vi "main.vi"() -> ()   [LabVIEW 2023]
panel:
  out "Fall Time":dbl format="%#_6ps"
  in  "Stop":bool
  in  "Start":bool
  out "Error_Out":errorcluster
  in  "Amplitude(V)":dbl=5.0
  out "Digital Signal":i32[](graph)
  out "Rise time":dbl format="%#_6ps"
  out "min value":dbl format="%#_3g V"
  out "max value":dbl format="%#_3g V"
  in  "Error_In":errorcluster
  out "Square Wave":waveform(dbl)(graph)={"t0"=timestamp(0 s since 1904-01-01), "dt"=1e-06, "Y"=array[5000 elements]}
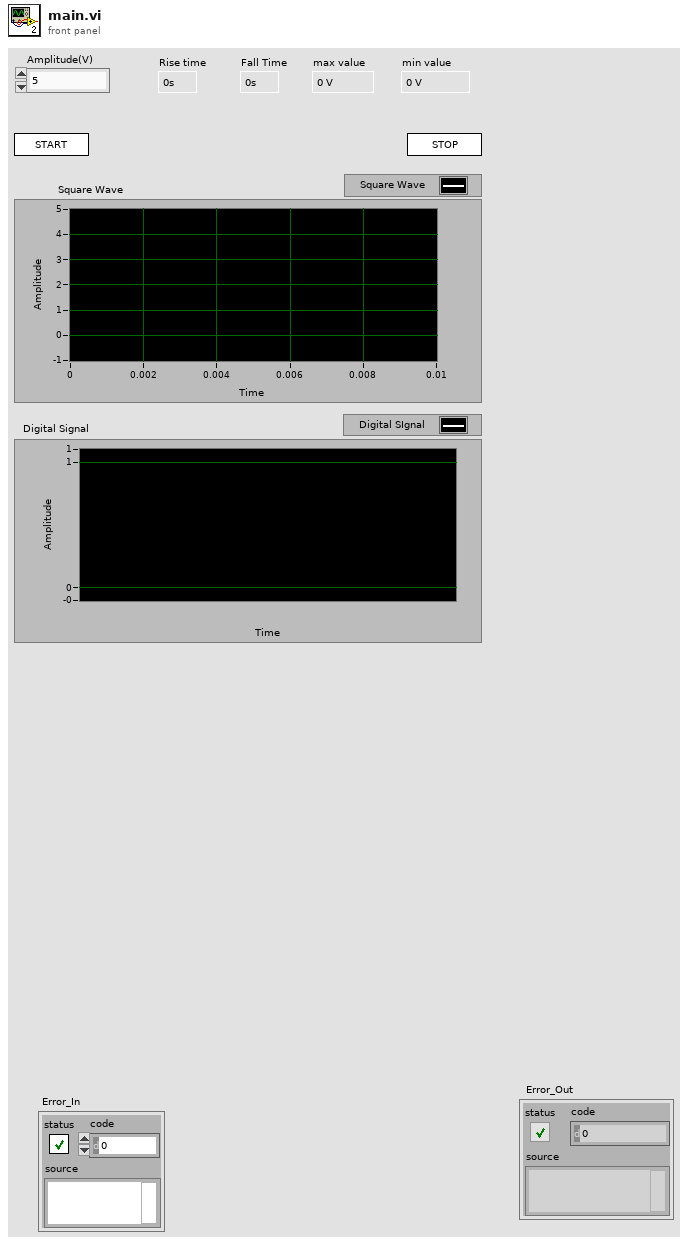
[diagram p1: front panel]
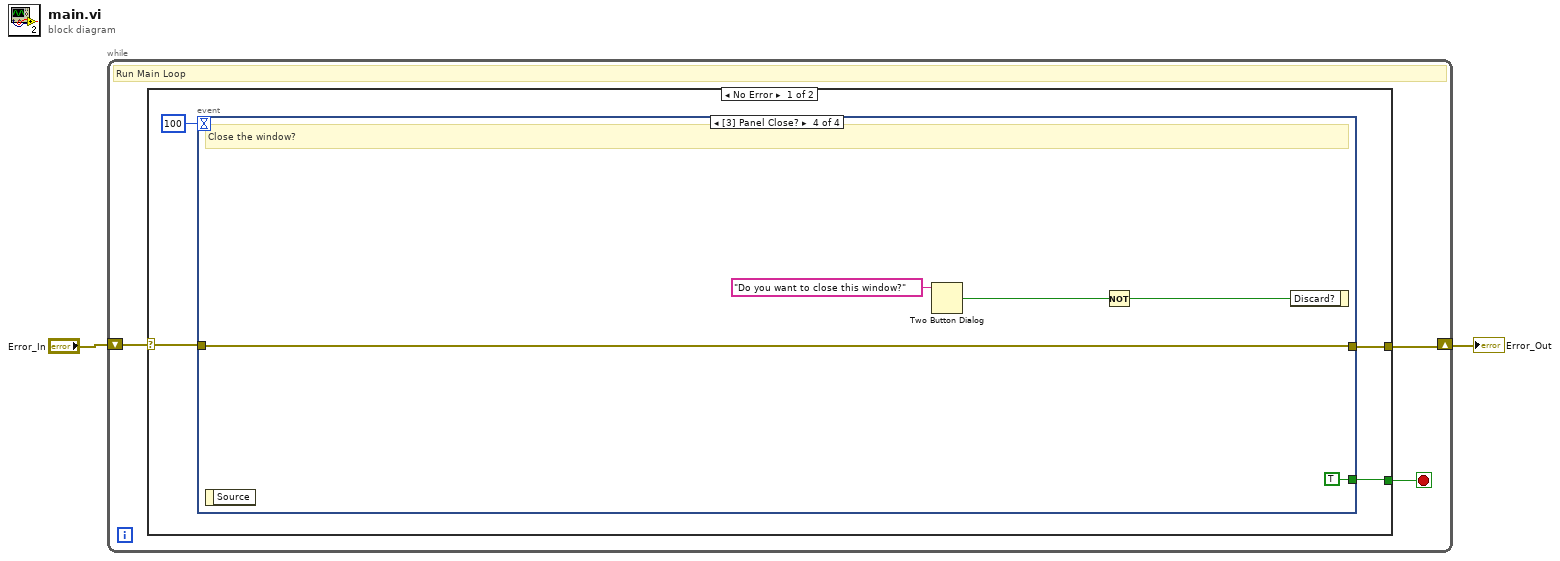
[diagram p0: block diagram]
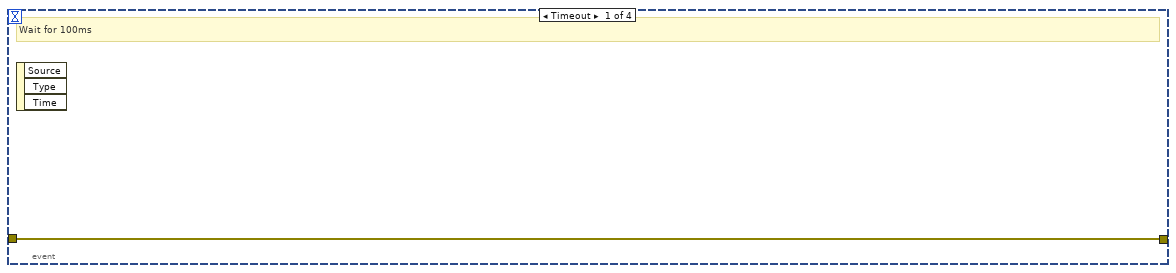
[diagram p2: hidden frame]
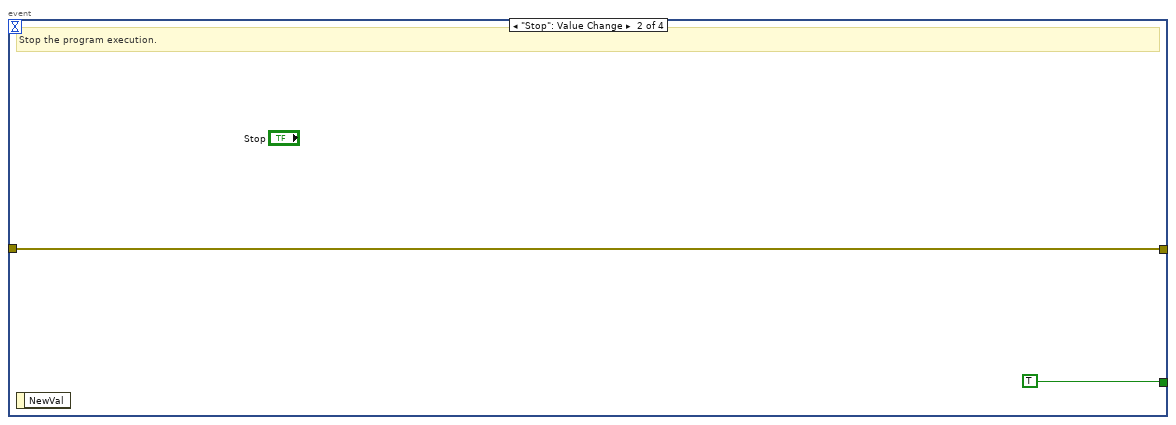
[diagram p3: hidden frame]
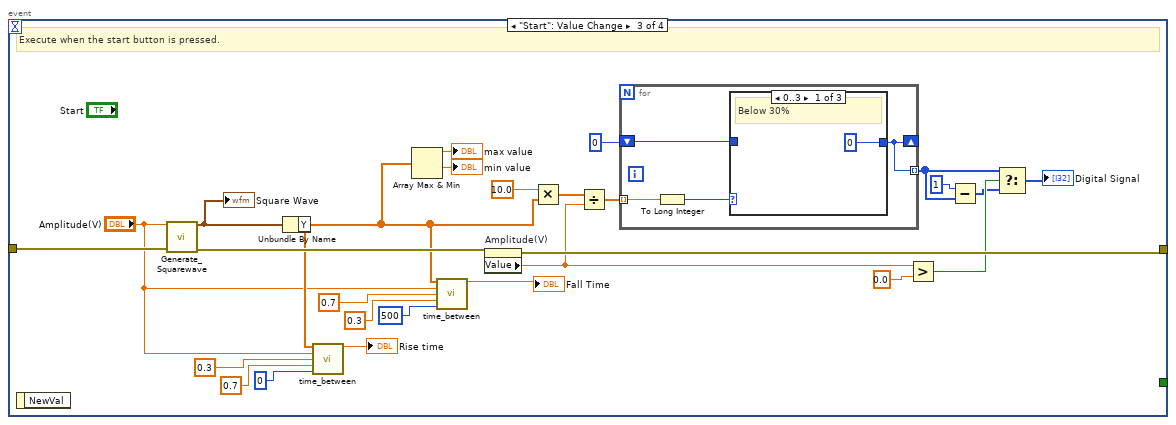
[diagram p4: hidden frame]
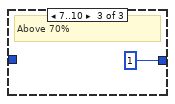
[diagram p6: hidden frame]
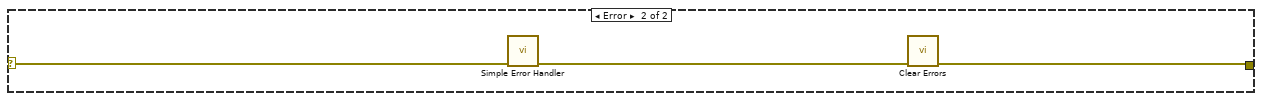
[diagram p7: hidden frame]
diagram:
  n1 = while {
    shift-right: [w3] -> w1
    shift-left: "Error_In" -> [w4]
    stop <- w5 stop-if-true
    # "Run Main Loop"
    n2 = case shown="No Error" w4 {
      selector: w4 -> [w7 w54]
      tunnel: [w8 _] -> w5
      tunnel: [w6 w52] -> w3
      frame No Error {
        n3 = event shown="[3] Panel Close?" {
          selector: _ -> [_ _ _ _]
          dyn-events: _ -> [_ _ _ _]
          timeout: 100 -> [_ _ _ _]
          tunnel: [_ TRUE _ TRUE] -> w8
          tunnel: w7 -> [w10 w11 w32 w51]
          tunnel: [w10 w11 w21 w51] -> w6
          event Timeout {
            # "Wait for 100ms"
            n4 = event-data() -> ()  [unwired: 1 in, 3 out]
          }
          event "Stop": Value Change {
            # "Stop the program execution."
            n5 = event-data() -> ()  [unwired: 1 in, 1 out]
          }
          event "Start": Value Change {
            # "Execute when the start button is pressed."
            n6 = event-data() -> ()  [unwired: 1 in, 1 out]
            n7 = call "Generate_Squarewave.vi"("Amplitude(V)"="Amplitude(V)", "Error_In"=w32) -> ("Waveform_Out"=w37:waveform(dbl), "Error_Out"=w30:errorcluster)  [unwired: 12 in]
            "Square Wave" <- w37
            n8 = Unbundle By Name(w37) -> ("Y"=w23:dbl[])
            n9 = call "time_between.vi"("Y"=w23, "Amplitude(V)"="Amplitude(V)", "First value"=0.3 ("y"), "Second Value"=0.7 ("x"), "index"=0) -> ("Numeric"=→"Rise time":dbl)  [unwired: 10 in]
            n10 = Array Max & Min(array=w23) -> (max value=→"max value":dbl, min value=→"min value":dbl)  [unwired: 2 out]
            n11 = call "time_between.vi"("Y"=w23, "Amplitude(V)"="Amplitude(V)", "First value"=0.7 ("y"), "Second Value"=0.3 ("x"), "index"=500) -> ("Numeric"=→"Fall Time":dbl)  [unwired: 10 in]
            n12 = property on="Amplitude(V)" class="DigNum (strict)"(error in=w30) -> (error out=w21:errorcluster, "Value"=w20:dbl)  [unwired: 1 in, 1 out]
            n13 = Multiply(x=10.0 ("y"), y=w23) -> (x*y=w31:dbl[])
            n14 = Divide(x=w31, y=w20) -> (x/y=w28:dbl[])
            n15 = for {
              shift-right: [w42] -> _
              shift-left: 0 -> [w43]
              tunnel: [w42] -> w15 mode=indexing
              tunnel: w28 -> [w41] mode=indexing
              n16 = To Long Integer(number=w41) -> (32bit integer=w40:i32)
              n17 = case shown="0..3" w40 {
                tunnel: w43 -> [_ w45 _]
                tunnel: [0 w45 1] -> w42
                frame 0..3 {
                  # "Below 30%"
                }
                frame 4..6, Default {
                  # "30-70%"
                }
                frame 7..10 {
                  # "Above 70%"
                }
              }
            }
            n18 = Greater?(x=w20, y=0.0) -> (0:w16:bool)
            n19 = Subtract(x=1, y=w15) -> (x-y=w14:i32[])
            n20 = Select(t=w15, s=w16, f=w14) -> (s? t:f=→"Digital Signal":i32[])
          }
          event Panel Close? {
            # "Close the window?"
            n21 = event-data() -> ()  [unwired: 1 in, 1 out]
            n22 = Two Button Dialog(message="Do you want to close this window?") -> (T button?=w50:bool)  [unwired: 2 in]
            n23 = Not(x=w50) -> (.not. x?=w49:bool)
            n24 = event-data("Discard?"=w49) -> ()  [unwired: 1 in, 1 out]
          }
        }
      }
      frame Error {
        n25 = call <vilib>:"Simple Error Handler.vi"("error in (no error)"=w54) -> ("error out"=w53:errorcluster)  [unwired: 4 in, 4 out]
        n26 = call <vilib>:"Clear Errors.vi"("error in (no error)"=w53) -> ("error out"=w52:errorcluster)  [unwired: 5 in, 1 out]
      }
    }
  }
  "Error_Out" <- w1
